vi "Reaction.vi"() -> ()   [LabVIEW 2017]
uses:
  61f5e3d0-52fd-49e3-84de-acee88744ddb.vi
  21a31181-54fe-4268-8d2e-5a6bfe5fdad5.vi
  1faa88df-fa28-4306-999d-8a34b3b41dda.vi
  a84fb1b2-72bc-4355-9d7d-0f2bfa19405c.vi
  d429babc-b0fa-4e1f-9f47-5200f57613f6.vi
  e025e46d-f501-4d92-95c5-4136c5052991.vi
  d631eef8-7fa0-41f0-9ac8-c450ba2948ee.vi
panel:
  in  "Stop Button":bool
  out "error out":errorcluster
  in  "error in (no error)":errorcluster
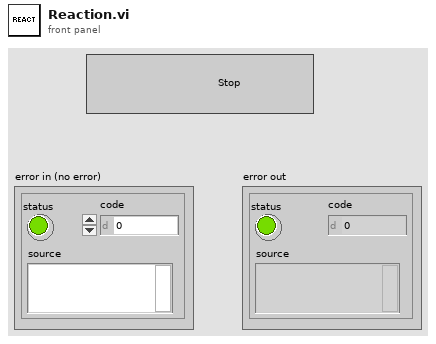
[diagram p1: front panel]
types:
  T1 = enum16{"off", "red", "green", "yellow", "blue", "pink", "cyan", "white"}
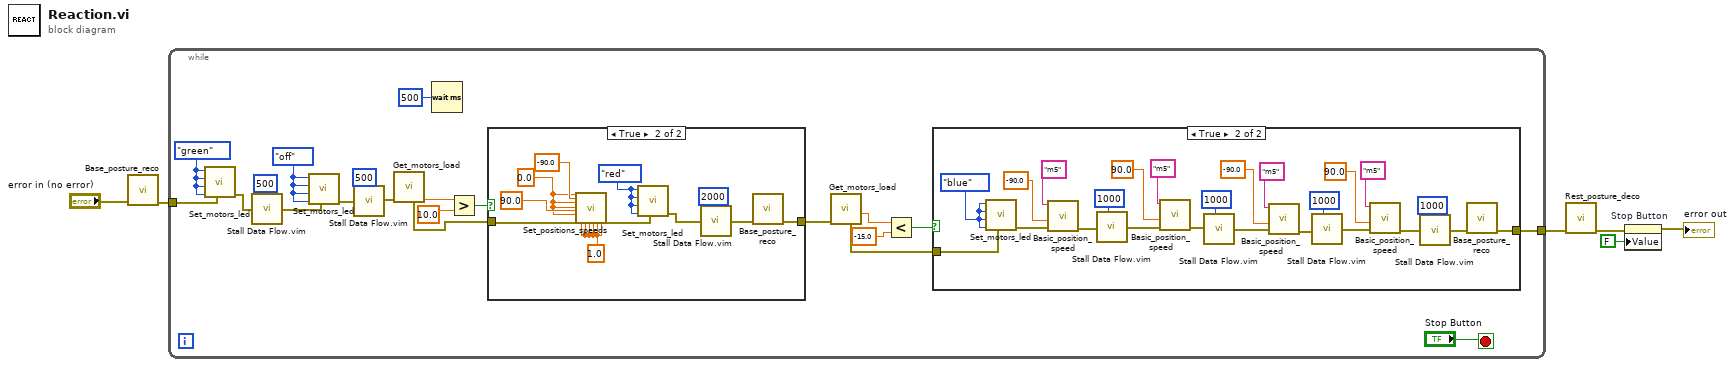
[diagram p0: block diagram]
diagram:
  n1 = call "Base_posture_reco.vi"("error in (no error)"="error in (no error)") -> ("error out"=w2:errorcluster)  [unwired: 10 in]
  n2 = while {
    tunnel: w2 -> [w8]
    tunnel: [w17] -> w1
    stop <- "Stop Button" stop-if-true
    w11 = T1."off" ("Color m2")
    w10 = T1."green" ("Color m2")
    n3 = call "Set_motors_led.vi"("error in (no error)"=w8, "Color m6"=w10, "Color m5"=w10, "Color m3"=w10, "Color m2"=w10) -> ("error out"=w14:errorcluster)  [unwired: 6 in]
    n4 = call "Stall Data Flow.vim"("value in"=w14, "milliseconds to wait"=u32 500) -> ("value out"=w16:errorcluster)  [unwired: 1 out]
    n5 = call "Set_motors_led.vi"("error in (no error)"=w16, "Color m6"=w11, "Color m5"=w11, "Color m3"=w11, "Color m2"=w11) -> ("error out"=w15:errorcluster)  [unwired: 6 in]
    n6 = call "Stall Data Flow.vim"("value in"=w15, "milliseconds to wait"=u32 500) -> ("value out"=w9:errorcluster)  [unwired: 1 out]
    n7 = call "Get_motors_load.vi"("error in (no error)"=w9) -> ("m6"=w27:dbl, "error out"=w20:errorcluster)  [unwired: 6 in, 3 out]
    n8 = Wait (ms)(milliseconds to wait=u32 500) -> ()  [unwired: 1 out]
    n9 = Greater?(x=w27, y=10.0) -> (0:w22:bool)
    n10 = case shown="True" w22 {
      tunnel: [w53 w54] -> w21
      tunnel: w20 -> [w53 w55]
      frame False {
      }
      frame True {
        w60 = T1."red" ("Color m2")
        w57 = 0.0 ("m1")
        w56 = 1.0 ("Speed m5")
        n11 = call "Set_positions_speeds.vi"("m1"=w57, "m2"=-90.0, "m3"=w57, "m4"=w57, "m5"=90.0, "m6"=w57, "error in (no error)"=w55, "Speed m1"=w56, "Speed m2"=w56, "Speed m3"=w56, "Speed m4"=w56, "Speed m5"=w56, "Speed m6"=w56) -> ("error out"=w61:errorcluster)  [unwired: 14 in]
        n12 = call "Set_motors_led.vi"("error in (no error)"=w61, "Color m6"=w60, "Color m5"=w60, "Color m3"=w60, "Color m2"=w60) -> ("error out"=w62:errorcluster)  [unwired: 6 in]
        n13 = call "Stall Data Flow.vim"("value in"=w62, "milliseconds to wait"=u32 2000) -> ("value out"=w64:errorcluster)  [unwired: 1 out]
        n14 = call "Base_posture_reco.vi"("error in (no error)"=w64) -> ("error out"=w54:errorcluster)  [unwired: 10 in]
      }
    }
    n15 = call "Get_motors_load.vi"("error in (no error)"=w21) -> ("m5"=w24:dbl, "error out"=w18:errorcluster)  [unwired: 6 in, 3 out]
    n16 = Less?(x=w24, y=-15.0) -> (x < y?=w19:bool)
    n17 = case shown="True" w19 {
      tunnel: w18 -> [w28 w47]
      tunnel: [w28 w46] -> w17
      frame False {
      }
      frame True {
        w50 = T1."blue" ("Color m2")
        n18 = call "Set_motors_led.vi"("error in (no error)"=w47, "Color m6"=w50, "Color m5"=w50, "Color m3"=w50, "Color m2"=w50) -> ("error out"=w45:errorcluster)  [unwired: 6 in]
        n19 = call "Basic_position_speed.vi"("error in (no error)"=w45, "Position m?"=-90.0, "m?"="m5") -> ("error out"=w44:errorcluster)  [unwired: 8 in]
        n20 = call "Stall Data Flow.vim"("value in"=w44, "milliseconds to wait"=u32 1000) -> ("value out"=w43:errorcluster)  [unwired: 1 out]
        n21 = call "Basic_position_speed.vi"("error in (no error)"=w43, "Position m?"=90.0, "m?"="m5") -> ("error out"=w42:errorcluster)  [unwired: 8 in]
        n22 = call "Stall Data Flow.vim"("value in"=w42, "milliseconds to wait"=u32 1000) -> ("value out"=w40:errorcluster)  [unwired: 1 out]
        n23 = call "Basic_position_speed.vi"("error in (no error)"=w40, "Position m?"=-90.0, "m?"="m5") -> ("error out"=w39:errorcluster)  [unwired: 8 in]
        n24 = call "Stall Data Flow.vim"("value in"=w39, "milliseconds to wait"=u32 1000) -> ("value out"=w38:errorcluster)  [unwired: 1 out]
        n25 = call "Basic_position_speed.vi"("error in (no error)"=w38, "Position m?"=90.0, "m?"="m5") -> ("error out"=w37:errorcluster)  [unwired: 8 in]
        n26 = call "Stall Data Flow.vim"("value in"=w37, "milliseconds to wait"=u32 1000) -> ("value out"=w49:errorcluster)  [unwired: 1 out]
        n27 = call "Base_posture_reco.vi"("error in (no error)"=w49) -> ("error out"=w46:errorcluster)  [unwired: 10 in]
      }
    }
  }
  n28 = call "Rest_posture_deco.vi"("error in (no error)"=w1) -> ("error out"=w4:errorcluster)  [unwired: 10 in]
  n29 = property on="Stop Button" class="Bool (strict)"(error in=w4, "Value"=FALSE ("Stop Button")) -> (error out=→"error out":errorcluster)  [unwired: 1 in, 1 out]
